vi "Mouse Hover.vi"(8 "error in (no error)":errorcluster, 10 "Coords":T1, 11 "MCListbox with Checkboxes in":refnum<class "MCListbox with Checkboxes.lvclass">) -> (0 "error out":errorcluster, 3 "MCListbox with Checkboxes out":refnum<class "MCListbox with Checkboxes.lvclass">)   [LabVIEW 2016, in "MCListbox with Checkboxes.lvclass"]
uses:
  MCListbox with Checkboxes.lvclass
  <vilib>/Utility/miscctls.llb/LVPoint32TypeDef.ctl
  MCListbox with Checkboxes.lvclass/MCListbox with Checkboxes.ctl
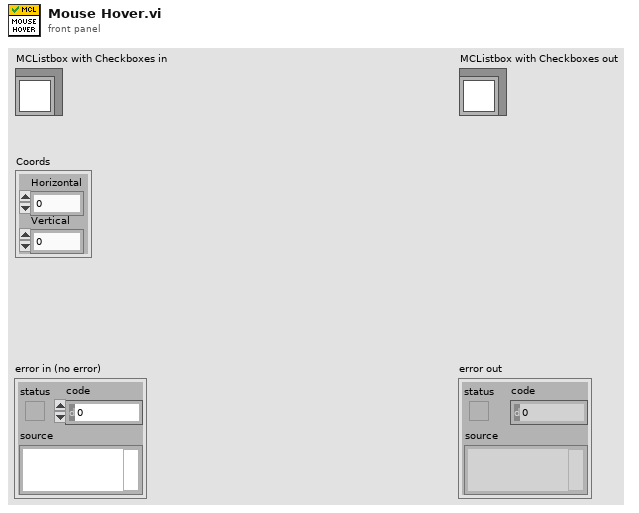
[diagram p1: front panel]
types:
  T1 = typedef "LVPoint32TypeDef.ctl" = cluster{"Horizontal":i32, "Vertical":i32}
  T2 = typedef "LVRowAndColumnTypeDef.ctl" = cluster{"Row":i32, "Column":i32}
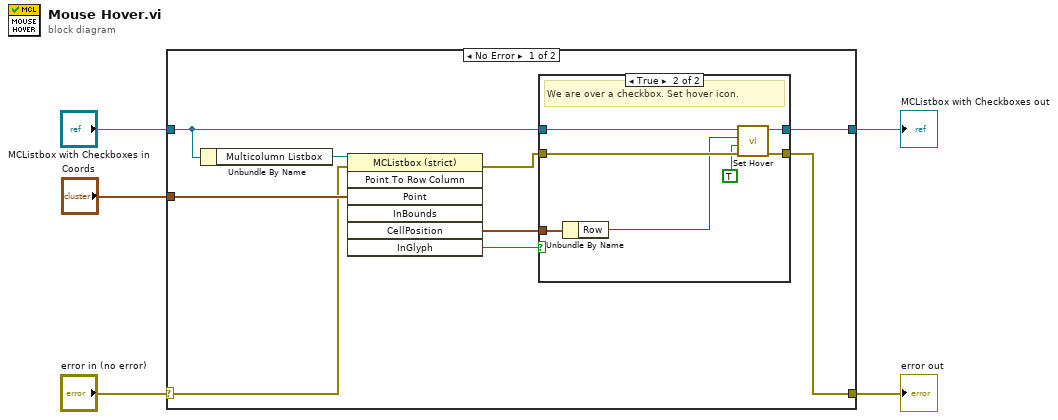
[diagram p0: block diagram]
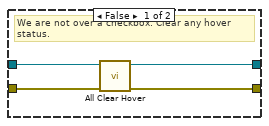
[diagram p2: hidden frame]
diagram:
  n1 = case shown="No Error" "error in (no error)" {
    selector: "error in (no error)" -> [w7 w27]
    tunnel: [w14 w27] -> w4
    tunnel: [w13 w26] -> w2
    tunnel: "MCListbox with Checkboxes in" -> [w12 w26]
    tunnel: "Coords" -> [w10 _]
    frame No Error {
      n2 = Unbundle By Name(w12) -> ("Multicolumn Listbox"=w11:refnum<vi>)
      n3 = invoke class="MCListbox (strict)" method="Point To Row Column"(reference=w11, error in=w7, "Point"=w10) -> (error out=w9:errorcluster, "CellPosition"=w6:T2, "InGlyph"=w8:bool)  [unwired: 4 in, 4 out]
      n4 = case shown="True" w8 {
        tunnel: w12 -> [w18 w25]
        tunnel: w9 -> [w17 w23]
        tunnel: [w16 w24] -> w13
        tunnel: [w15 w21] -> w14
        tunnel: w6 -> [_ w20]
        frame False {
          # "We are not over a checkbox. Clear any hover status."
          n5 = call "All Clear Hover.vi"("error in (no error)"=w17, "MCListbox with Checkboxes in"=w18) -> ("error out"=w15:errorcluster, "MCListbox with Checkboxes out"=w16:refnum<class "MCListbox with Checkboxes.lvclass">)  [unwired: 8 in]
        }
        frame True {
          # "We are over a checkbox. Set hover icon."
          n6 = Unbundle By Name(w20) -> ("Row"=w19:i32)
          n7 = call "Set Hover.vi"("error in (no error)"=w23, "Set Hover (F)"=TRUE, "Index"=w19, "MCListbox with Checkboxes in"=w25) -> ("error out"=w21:errorcluster, "MCListbox with Checkboxes out"=w24:refnum<class "MCListbox with Checkboxes.lvclass">)  [unwired: 6 in]
        }
      }
    }
    frame Error {
    }
  }
  "error out" <- w4
  "MCListbox with Checkboxes out" <- w2
